vi "Protocol.RQST Wait on Multiple Requests.vi"(6 "Processed Outgoing":refnum<queue>, 7 "Name":string, 8 "error in (no error)":errorcluster, 9 "value":T4[](array[typedef]), 10 "Source Address":u8=27, 11 "ref in":T3) -> (0 "error out":errorcluster, 1 "Global Requests":bool[](array[boolean]), 2 "Timeouts":bool[](array[boolean]), 3 "Elements":T1[](array[typedef]) {"payload" format="%x"; "timestamp" format="%<%.7X\n%x>T"; "type" items=["CAN Data"=0, "CAN Remote"=1, "CAN Bus Error"=2, "CAN 2.0 Data"=8, "CAN FD Data"=16, "CAN FD+BRS Data"=24, "J1939 Data"=192, "Delay"=224, "Log Trigger"=225, "Start Trigger"=226]; "identifier" format="%x"}, 5 "Ignore Response?":bool)   [LabVIEW 2023, in "J1939 Addon Engine.lvlib"]
uses:
  J1939 Addon Engine.lvlib
  Addon Shared/Types/Request Message.ctl
  Types/Protocol.RQST Lookup Table Reference.ctl
  <vilib>/xnet/xnet.llb/XNET Frame CAN.ctl
  <vilib>/xnet/xnet.llb/XNET Frame Type CAN.ctl
  Support Libraries/J1939 Utilities/Types/CAN Outgoing Message Cluster.ctl
  Types/Protocol.RQST Lookup Table Action.ctl
  Types/Protocol.RQST Lookup Table Cluster.ctl
  Support Libraries/J1939 Utilities/SubVIs/Request.vi
  Support Libraries/J1939 Utilities/Common Conversions.vi
  Support Libraries/J1939 Utilities/SubVIs/Convert J1939 ID to CAN Arb ID.vi
  Protocol.RQST Lookup Table.vi
  Support Libraries/J1939 Utilities/J1939 Utilities.lvlib
  Addon Shared/J1939 Addon Shared.lvlib
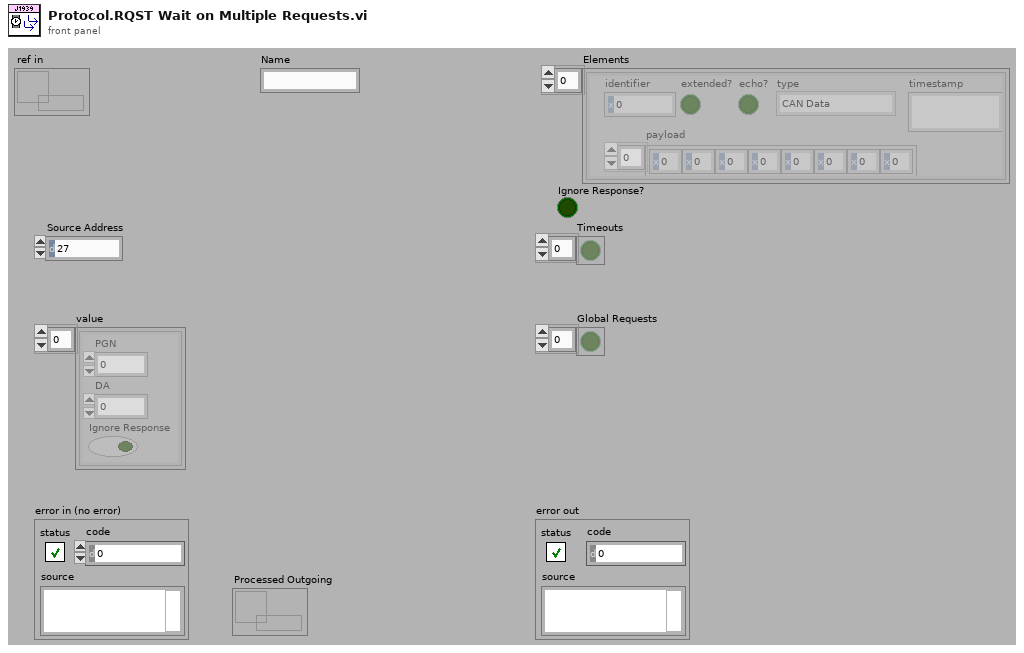
[diagram p1: front panel]
types:
  T1 = typedef "XNET Frame CAN.ctl" = cluster{"timestamp":timestamp, "payload":u8[], "identifier":u32, "type":T2, "extended?":bool, "echo?":bool}
  T2 = typedef "XNET Frame Type CAN.ctl" = u8
  T3 = typedef "J1939 Addon Engine.lvlib/Protocol.RQST Lookup Table Reference.ctl" = refnum<data-value>
  T4 = typedef "J1939 Addon Shared.lvlib/Request Message.ctl" = cluster{"PGN":u32, "DA":u8, "Ignore Response":bool}
  T5 = typedef "J1939 Addon Engine.lvlib/Protocol.RQST Lookup Table Action.ctl" = enum16{"Initialize", "Add", "Get", "Remove", "Get Active Requests"}
  T6 = typedef "J1939 Utilities.lvlib/CAN Outgoing Message Cluster.ctl" = cluster{"Identifier":u32, "Data":u8[]}
  T7 = typedef "J1939 Addon Engine.lvlib/Protocol.RQST Lookup Table Cluster.ctl" = cluster{"Response Q":refnum<queue>, "Request PGN":u32}
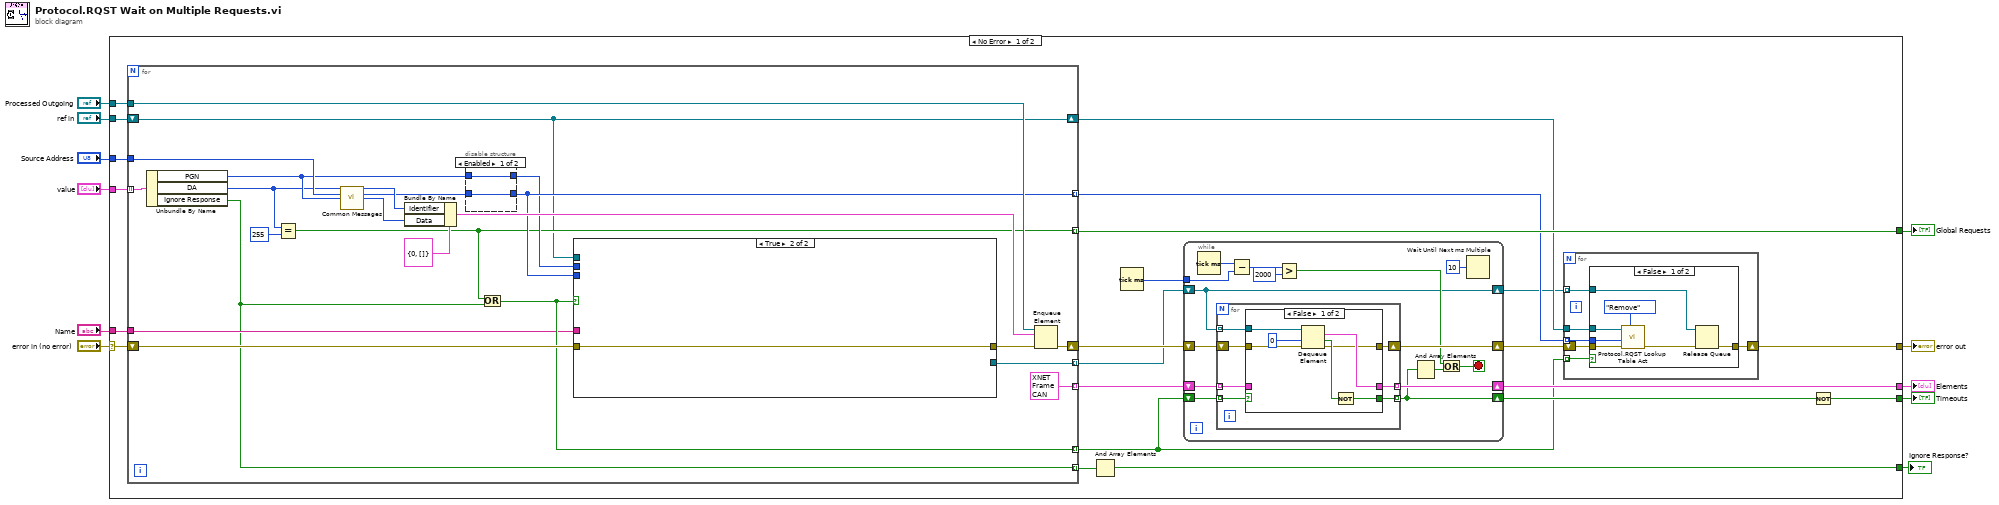
[diagram p0: block diagram]
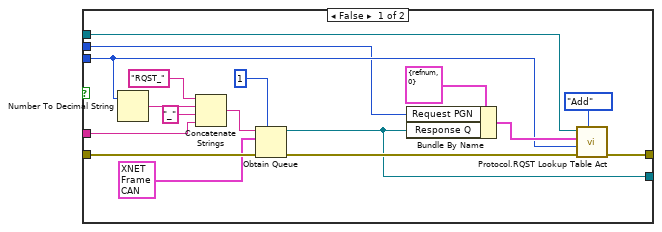
[diagram p4: hidden frame]
diagram:
  n1 = case shown="No Error" "error in (no error)" {
    selector: "error in (no error)" -> [w33 w124]
    tunnel: "Source Address" -> [w28 _]
    tunnel: "ref in" -> [w20 _]
    tunnel: [w23 w124] -> w7
    tunnel: [w32 _] -> w9
    tunnel: [w18 _] -> w8
    tunnel: "Processed Outgoing" -> [w29 _]
    tunnel: [w27 _] -> w4
    tunnel: "value" -> [w26 _]
    tunnel: "Name" -> [w14 _]
    tunnel: [w12 _] -> w1
    frame No Error {
      n2 = for {
        tunnel: [w101] -> w16 mode=indexing
        tunnel: w29 -> [w98]
        tunnel: [w92] -> w22 mode=indexing
        tunnel: w28 -> [w90]
        tunnel: [w88] -> w19 mode=indexing
        tunnel: [w87] -> w27 mode=indexing
        shift-right: [w99] -> w30
        shift-left: w33 -> [w102]
        tunnel: w26 -> [w86] mode=indexing
        shift-right: [w83] -> w21
        shift-left: w20 -> [w83]
        tunnel: [T1 {"timestamp"=timestamp(0 s since 1904-01-01), "payload"=[], "identifier"=0, "type"=0, "extended?"=FALSE, "echo?"=FALSE} ("CAN frame")] -> w15 mode=indexing
        tunnel: w14 -> [w81]
        tunnel: [w80] -> w13 mode=indexing
        n3 = Unbundle By Name(w86) -> ("PGN"=w85:u32, "DA"=w84:u8, "Ignore Response"=w80:bool)
        n4 = Equal?(x=w84, y=u8 255) -> (x = y?=w87:bool)
        n5 = call-poly "Common Messages.vi"("Destination Address"=w84, "Source Address"=w90, "PGN"=w85) -> ("Arb ID"=w95:u32, "Expected Return Arb ID"=w93:u32, "Data"=w96:u8[])  [unwired: 10 in]
        n6 = Bundle By Name(cluster=T6 {"Identifier"=0, "Data"=[]} ("element"), "Identifier"=w95, "Data"=w96) -> (w94:T6)
        n7 = disable-structure shown="Enabled" {
          disable-tunnel: [w122 w123] -> w92
          disable-tunnel: w93 -> [w122 _]
          disable-tunnel: w85 -> [w121 w123]
          disable-tunnel: [w121 w123] -> w91
          frame Enabled {
          }
          frame Disabled {
          }
        }
        n8 = Or(x=w87, y=w80) -> (x .or. y?=w88:bool)
        n9 = case shown="True" w88 {
          tunnel: w102 -> [w118 w120]
          tunnel: w83 -> [w113 _]
          tunnel: [w112 _] -> w101
          tunnel: [w111 w120] -> w100
          tunnel: w92 -> [w105 _]
          tunnel: w91 -> [w104 _]
          tunnel: w81 -> [w108 _]
          frame False {
            n10 = Number To Decimal String(number=w105) -> (decimal integer string=w106:string)  [unwired: 1 in]
            n11 = Concatenate Strings("RQST_" ("string"), w106, "_" ("string"), w108) -> (w107:string)
            n12 = Obtain Queue(max queue size (-1, unlimited)=1, name (unnamed)=w107, element data type=T1 {"timestamp"=timestamp(0 s since 1904-01-01), "payload"=[], "identifier"=0, "type"=0, "extended?"=FALSE, "echo?"=FALSE} ("CAN frame"), error in (no error)=w118) -> (queue out=w112:refnum<queue>, error out=w117:errorcluster)  [unwired: 1 in, 1 out]
            n13 = Bundle By Name(cluster=T7 {"Response Q"=refnum, "Request PGN"=0} ("Data"), "Request PGN"=w104, "Response Q"=w112) -> (w114:T7)
            n14 = call "Protocol.RQST Lookup Table Act.vi"("Action"=Protocol.RQST_Lookup_Table_Action."Add", "error in (no error)"=w117, "ID"=w105, "Data"=w114, "Rqst LUT"=w113) -> ("error out"=w111:errorcluster)  [unwired: 2 in, 4 out]
          }
          frame True {
          }
        }
        n15 = Enqueue Element(queue=w98, element=w94, error in (no error)=w100) -> (error out=w99:errorcluster)  [unwired: 1 in, 2 out]
      }
      n16 = And Array Elements(Boolean array=w13) -> (logical AND=w12:bool)
      n17 = Tick Count (ms)() -> (millisecond timer value=w25:u32)
      n18 = while {
        shift-right: [w61] -> w32
        shift-left: w15 -> [w58]
        shift-right: [w57] -> w31
        shift-left: w19 -> [w59]
        tunnel: w25 -> [w53]
        shift-right: [w62] -> w24
        shift-left: w30 -> [w60]
        shift-right: [w49] -> w17
        shift-left: w16 -> [w49]
        stop <- w55 stop-if-true
        n19 = Tick Count (ms)() -> (millisecond timer value=w54:u32)
        n20 = for {
          tunnel: w49 -> [w69] mode=indexing
          tunnel: [w67] -> w61 mode=indexing
          tunnel: [w66] -> w57 mode=indexing
          tunnel: w59 -> [w64] mode=indexing
          tunnel: w58 -> [w63] mode=indexing
          shift-right: [w68] -> w62
          shift-left: w60 -> [w65]
          n21 = case shown="False" w64 {
            selector: w64 -> [_ w78]
            tunnel: w69 -> [w75 _]
            tunnel: [w71 w79] -> w68
            tunnel: [w74 w77] -> w67
            tunnel: [w70 w78] -> w66
            tunnel: w65 -> [w72 w79]
            tunnel: w63 -> [_ w77]
            frame False {
              n22 = Dequeue Element(queue=w75, timeout in ms (-1)=0, error in (no error)=w72) -> (element=w74:T1, timed out?=w73:bool, error out=w71:errorcluster)  [unwired: 1 out]
              n23 = Not(x=w73) -> (.not. x?=w70:bool)
            }
            frame True {
            }
          }
        }
        n24 = Subtract(x=w54, y=w53) -> (x-y=w52:u32)
        n25 = Greater?(x=w52, y=u32 2000) -> (0:w50:bool)
        n26 = And Array Elements(Boolean array=w57) -> (logical AND=w56:bool)
        n27 = Or(x=w50, y=w56) -> (x .or. y?=w55:bool)
        n28 = Wait Until Next ms Multiple(millisecond multiple=u32 10) -> ()  [unwired: 1 out]
      }
      n29 = for {
        shift-right: [w38] -> w23
        shift-left: w24 -> [w39]
        tunnel: w17 -> [w37] mode=indexing
        tunnel: w22 -> [w36] mode=indexing
        tunnel: w21 -> [w35]
        tunnel: w19 -> [w34] mode=indexing
        n30 = case shown="False" w34 {
          tunnel: w35 -> [w46 _]
          tunnel: [w44 w47] -> w38
          tunnel: w39 -> [w41 w47]
          tunnel: w36 -> [w43 _]
          tunnel: w37 -> [w42 _]
          frame False {
            n31 = call "Protocol.RQST Lookup Table Act.vi"("Action"=Protocol.RQST_Lookup_Table_Action."Remove", "error in (no error)"=w41, "ID"=w43, "Rqst LUT"=w46) -> ("error out"=w45:errorcluster)  [unwired: 3 in, 4 out]
            n32 = Release Queue(queue=w42, error in (no error)=w45) -> (error out=w44:errorcluster)  [unwired: 1 in, 2 out]
          }
          frame True {
          }
        }
      }
      n33 = Not(x=w31) -> (.not. x?=w18:bool[])
    }
    frame Error {
    }
  }
  "Elements" <- w9
  "Timeouts" <- w8
  "error out" <- w7
  "Global Requests" <- w4
  "Ignore Response?" <- w1
